vi "InsertNewRequest.vi"(8 "error in":errorcluster, 11 "Request.lvclass":refnum<class "Request.lvclass">) -> (0 "error out":errorcluster, 3 "Request out":refnum<class "Request.lvclass">)   [LabVIEW 2015, in "DatabaseApi.lvlib"]
uses:
  DatabaseApi.lvlib
  LVClasses/Request/Request.lvclass
  TypeDef/Request/RequestsTableDbTableName.ctl
  TypeDef/Request/RequestsTableColumnNames.ctl
  LVClasses/Request/Request.lvclass/Request.ctl
  LVClasses/Request/RequestCluster.ctl
  LVClasses/Request/PersonnelType.ctl
  LVClasses/Request/RequestType.ctl
  <vilib>/addons/database/Connection.llb/DB Tools Open Connec (String).vi
  <vilib>/addons/database/NI_Database_API.lvlib
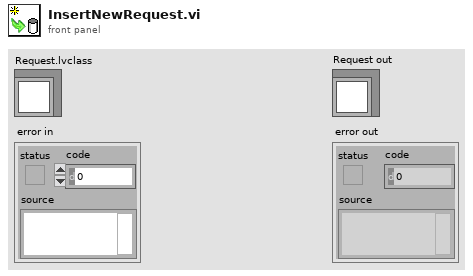
[diagram p1: front panel]
types:
  T1 = typedef "DatabaseApi.lvlib/RequestsTableColumnNames.ctl" = string[]
  T2 = typedef "DatabaseApi.lvlib/RequestsTableDbTableName.ctl" = string
  T3 = typedef "Request.lvclass/PersonnelType.ctl" = u16
  T4 = typedef "Request.lvclass/RequestType.ctl" = enum16{"Specific Call To Room", "General Call To Room"}
  T5 = typedef "Request.lvclass/RequestCluster.ctl" = cluster{"RequestID":string, "PersonelType":T3, "StartTime":timestamp, "StartName":string, "AckTime":timestamp, "AckName":string, "FulfilledTime":timestamp, "FulfilledName":string, "Description":string, "Room Number":i32, "Request Type":T4, "Alarm":bool}
  T6 = typedef "NI_Database_API.lvlib/Conn ObjectReference.ctl" = refnum<k1>
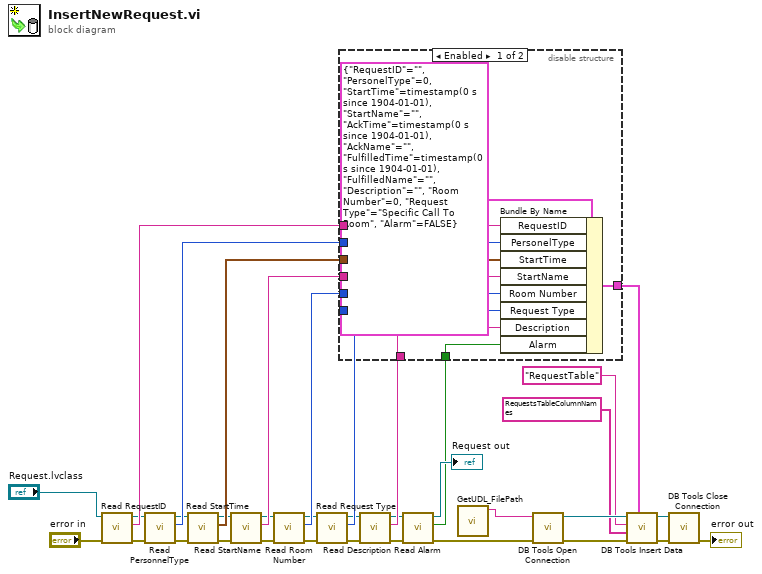
[diagram p0: block diagram]
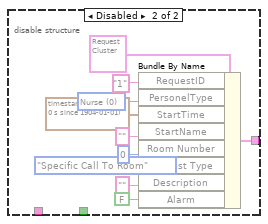
[diagram p2: hidden frame]
diagram:
  n1 = call "Read RequestID.vi"("error in (no error)"="error in", "Request in"="Request.lvclass") -> ("error out"=w24:errorcluster, "RequestID"=w26:string, "Request out"=w23:refnum<class "Request.lvclass">)  [unwired: 7 in]
  n2 = call "Read PersonnelType.vi"("error in (no error)"=w24, "Request in"=w23) -> ("error out"=w21:errorcluster, "PersonnelType"=w22:T3, "Request out"=w20:refnum<class "Request.lvclass">)  [unwired: 7 in]
  n3 = call "Read StartTime.vi"("error in (no error)"=w21, "Request in"=w20) -> ("error out"=w18:errorcluster, "StartTime"=w19:timestamp, "Request out"=w17:refnum<class "Request.lvclass">)  [unwired: 7 in]
  n4 = call "Read StartName.vi"("error in (no error)"=w18, "Request in"=w17) -> ("error out"=w15:errorcluster, "StartName"=w16:string, "Request out"=w14:refnum<class "Request.lvclass">)  [unwired: 7 in]
  n5 = call "Read Room Number.vi"("error in (no error)"=w15, "Request in"=w14) -> ("error out"=w12:errorcluster, "Room Number"=w13:i32, "Request out"=w11:refnum<class "Request.lvclass">)  [unwired: 7 in]
  n6 = call "Read Request Type.vi"("error in (no error)"=w12, "Request in"=w11) -> ("error out"=w9:errorcluster, "Request Type"=w10:T4, "Request out"=w8:refnum<class "Request.lvclass">)  [unwired: 7 in]
  n7 = call "Read Description.vi"("error in (no error)"=w9, "Request in"=w8) -> ("error out"=w6:errorcluster, "Description"=w7:string, "Request out"=w3:refnum<class "Request.lvclass">)  [unwired: 7 in]
  n8 = call "Read Alarm.vi"("error in (no error)"=w6, "Request in"=w3) -> ("error out"=w4:errorcluster, "Alarm"=w1:bool, "Request out"=→"Request out":refnum<class "Request.lvclass">)  [unwired: 7 in]
  n9 = disable-structure shown="Enabled" {
    disable-tunnel: [w45 w55] -> w28
    disable-tunnel: w26 -> [w43 _]
    disable-tunnel: w22 -> [w42 _]
    disable-tunnel: w19 -> [w41 _]
    disable-tunnel: w16 -> [w40 _]
    disable-tunnel: w13 -> [w39 _]
    disable-tunnel: w10 -> [w38 _]
    disable-tunnel: w7 -> [w37 _]
    disable-tunnel: w1 -> [w36 _]
    frame Enabled {
      n10 = Bundle By Name(cluster=T5 {"RequestID"="", "PersonelType"=0, "StartTime"=timestamp(0 s since 1904-01-01), "StartName"="", "AckTime"=timestamp(0 s since 1904-01-01), "AckName"="", "FulfilledTime"=timestamp(0 s since 1904-01-01), "FulfilledName"="", "Description"="", "Room Number"=0, "Request Type"=enum."Specific Call To Room", "Alarm"=FALSE} ("RequestTable"), "RequestID"=w43, "PersonelType"=w42, "StartTime"=w41, "StartName"=w40, "Room Number"=w39, "Request Type"=w38, "Description"=w37, "Alarm"=w36) -> (w45:T5)
    }
    frame Disabled {
      w52 = T3 0 items=["Nurse", "Doctor", "Cleanning", "Admin"] ("PersonelType")
      n11 = Bundle By Name(cluster=T5 {"RequestID"="", "PersonelType"=0, "StartTime"=timestamp(0 s since 1904-01-01), "StartName"="", "AckTime"=timestamp(0 s since 1904-01-01), "AckName"="", "FulfilledTime"=timestamp(0 s since 1904-01-01), "FulfilledName"="", "Description"="", "Room Number"=0, "Request Type"=enum."Specific Call To Room", "Alarm"=FALSE} ("RequestTable"), "RequestID"="1", "PersonelType"=w52, "StartTime"=timestamp(3562278180 s since 1904-01-01), "StartName"="", "Room Number"=0, "Request Type"=RequestType."Specific Call To Room", "Description"="", "Alarm"=FALSE) -> (w55:T5)
    }
  }
  n12 = call "GetUDL_FilePath.vi"() -> ("UDL file path"=w35:string)  [unwired: 11 in]
  n13 = call-poly <vilib>:"DB Tools Open Connection.vi"("error in (no error)"=w4, "connection information"=w35) -> ("error out"=w31:errorcluster, "connection reference"=w32:T6)  [unwired: 6 in]
  n14 = call <vilib>:"DB Tools Insert Data.vi"("data"=w28, "error in (no error)"=w31, "columns"=T1 ["RequestID", "PersonnelType", "StartTime", "StartName", "AckTime", "AckName", "FulfilledTime", "FulfilledName", "Description", "RoomNumber", "RequestType", "Alarm"] ("Array"), "table"=T2 "RequestTable" ("RequestTable"), "connection reference"=w32) -> ("error out"=w33:errorcluster, "connection reference out"=w34:T6)  [unwired: 5 in]
  n15 = call <vilib>:"DB Tools Close Connection.vi"("error in (no error)"=w33, "connection reference"=w34) -> ("error out"=→"error out":errorcluster)  [unwired: 5 in]
